vi "Class_Tree Tag_Encode.vi"(7 "Action":T2=enum."In Place Reorder", 8 "Property Type":T1(ring), 9 "Index":u16, 10 "Hierarchy":string, 11 "Unique ID string":string) -> (0 "Parents":string[](array[string]), 1 "Indent":i32, 2 "Tag":string, 3 "Display name":string)   [LabVIEW 2023]
doc: "By using the long name localized for the tag, children of search matches will be shown. ID is required in tag bc we set the property node terminals by ID.\n\nThe display value will be the short name for property and method dialogs, and the full name for remove and rearrange dialongs.\n\nFormat is\n\nindex.propertyType.parent:shortName where parent:shortName=Long name (localized)\n\nAll properties classses and methods have a property item which contains the class/property heirarchy in a colon delimited list. This is used in sorting and filtering of items."
uses:
  controls/action enum.ctl
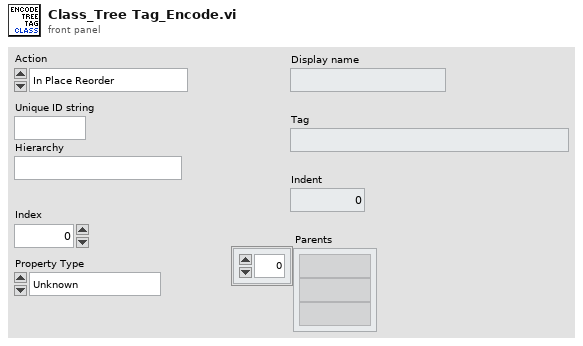
[diagram p1: front panel]
types:
  T1 = enum16{"Unknown", "Base", "Scripting", "Private", "Deprecated"}
  T2 = typedef "action enum.ctl" = enum16{"[NONE]", "APP_SEPARATOR", "Wire Bundle", "Wire Unbundle", "Terminal Unbundle", "Terminal Bundle", "Bundler Move Up", "Bundler Move Down", "Bundler Insert", "Bundler Remove", "Bundler Remove Unwired", "Bundler Reorder", "In Place Insert", "In Place Remove", "In Place Remove Unwired", "In Place Reorder", "Wire Properties", "Wire Method", "Terminal Properties", "Terminal Method", "Property Move Up", "Property Move Down", "Properties Insert", "Properties Remove", "Properties Remove Unwired", "Properties Reorder", "Method Change", "Class For Constant", "Class For Control", "Class For Node", "Class Name to Clipboard"}
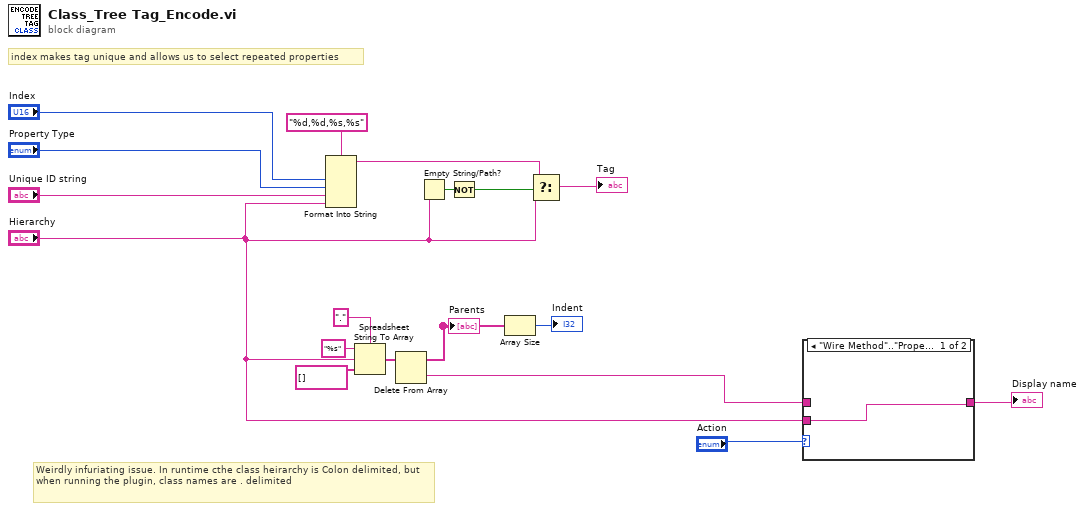
[diagram p0: block diagram]
diagram:
  # "Weirdly infuriating issue. In runtime cthe class heirarchy is Colon delimited, but when running the plugin, class names are . delimited"
  # "index makes tag unique and allows us to select repeated properties"
  n1 = Format Into String(format string="%d,%d,%s,%s", "Index", "Property Type", "Unique ID string", "Hierarchy") -> (resulting string=w17:string)  [unwired: 2 in, 1 out]
  n2 = Spreadsheet String To Array(delimiter (Tab)=".", format string="%s", spreadsheet string="Hierarchy", array type (2D Dbl)=string[] []) -> (array=w7:string[])
  n3 = Delete From Array(array=w7) -> (deleted portion=w3:string, array with subset deleted=w6:string[])  [unwired: 2 in]
  "Parents" <- w6
  n4 = Empty String/Path?(string/path="Hierarchy") -> (empty?=w15:bool)
  n5 = Not(x=w15) -> (.not. x?=w14:bool)
  n6 = Array Size(array=w6) -> (size(s)=→"Indent":i32)
  n7 = Select(t=w17, s=w14, f="Hierarchy") -> (s? t:f=→"Tag":string)
  n8 = case shown="\"Wire Method\"..\"Properties Remove\"" "Action" {
    tunnel: [w19 w20] -> w4
    tunnel: w3 -> [_ w20]
    tunnel: "Hierarchy" -> [w19 _]
    frame "Wire Method".."Properties Remove" {
    }
    frame Default {
    }
  }
  "Display name" <- w4
